vi "Equals.vi"(8 "error in (no error)":errorcluster, 10 "Other Parameter to Hardware Map in":refnum<class "Parameter to Hardware Map.lvclass">, 11 "Parameter to Hardware Map in":refnum<class "Parameter to Hardware Map.lvclass">) -> (0 "error out":errorcluster, 2 "Equal?":bool, 3 "Parameter to Hardware Map out":refnum<class "Parameter to Hardware Map.lvclass">)   [LabVIEW 2020, in "Parameter to Hardware Map.lvclass"]
doc: "Test if two maps are equal. Item order is not considered. Maps are considered equal if all elements of map_1 are included in map_2 and all elements of map_2 are included in map_1."
uses:
  Parameter to Hardware Map.lvclass
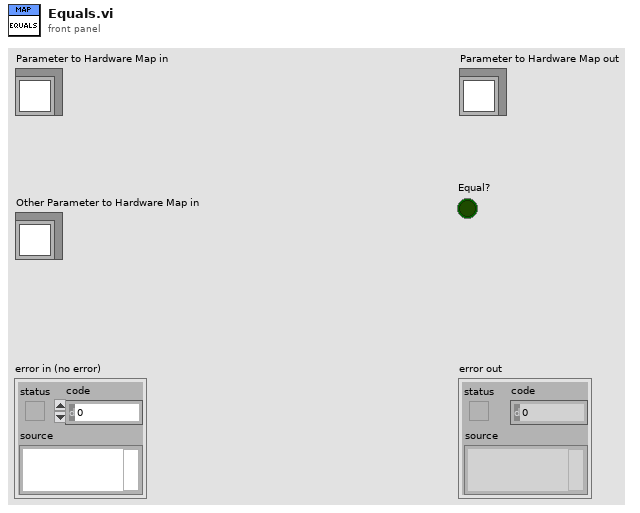
[diagram p1: front panel]
types:
  T1 = typedef "Parameter to Hardware Map.lvclass/Pair.ctl" = cluster{"key":string, "values":refnum<class "Generic Plugin.lvclass">[]}
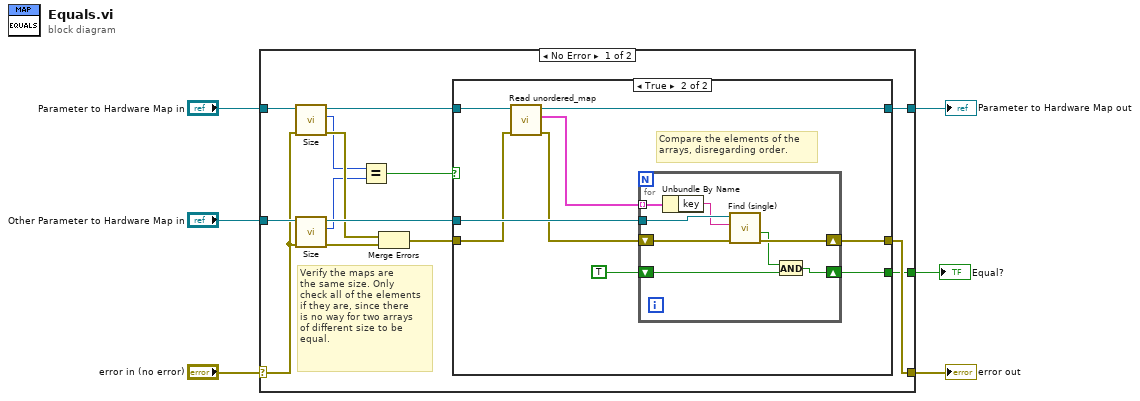
[diagram p0: block diagram]
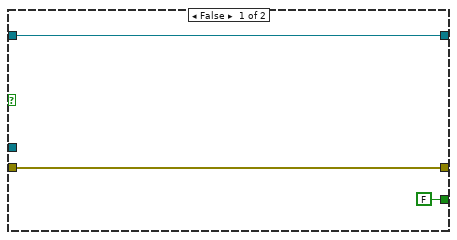
[diagram p2: hidden frame]
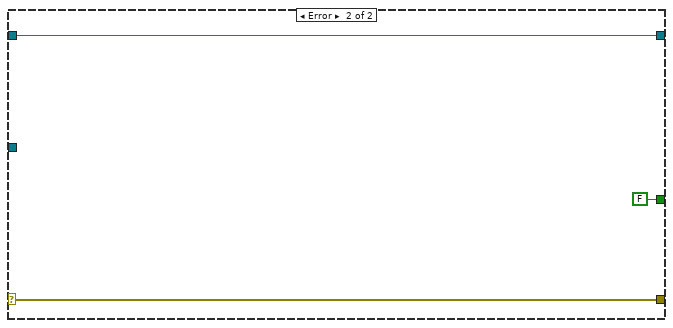
[diagram p3: hidden frame]
diagram:
  n1 = case shown="No Error" "error in (no error)" {
    selector: "error in (no error)" -> [w14 w43]
    tunnel: [w18 w43] -> w5
    tunnel: [w19 w42] -> w3
    tunnel: "Parameter to Hardware Map in" -> [w20 w42]
    tunnel: "Other Parameter to Hardware Map in" -> [w17 _]
    tunnel: [w7 FALSE] -> w1
    frame No Error {
      # "Verify the maps are\nthe same size. Only\ncheck all of the elements\nif they are, since there\nis no way for two arrays\nof different size to be\nequal."
      n2 = call "Size.vi"("error in (no error)"=w14, "Parameter to Hardware Map in"=w20) -> ("error out"=w12:errorcluster, "Size"=w11:i32, "Parameter to Hardware Map out"=w16:refnum<class "Parameter to Hardware Map.lvclass">)  [unwired: 7 in]
      n3 = call "Size.vi"("error in (no error)"=w14, "Parameter to Hardware Map in"=w17) -> ("error out"=w13:errorcluster, "Size"=w10:i32, "Parameter to Hardware Map out"=w15:refnum<class "Parameter to Hardware Map.lvclass">)  [unwired: 7 in]
      n4 = Equal?(x=w11, y=w10) -> (x = y?=w8:bool)
      n5 = Merge Errors(w12, w13) -> (w9:errorcluster)
      n6 = case shown="True" w8 {
        tunnel: [w23 w32] -> w19
        tunnel: [w22 w30] -> w18
        tunnel: w16 -> [w23 w28]
        tunnel: w15 -> [_ w27]
        tunnel: w9 -> [w22 w26]
        tunnel: [FALSE w24] -> w7
        frame False {
        }
        frame True {
          # "Compare the elements of the \narrays, disregarding order."
          n7 = call "Read unordered_map.vi"("error in (no error)"=w26, "Parameter to Hardware Map in"=w28) -> ("error out"=w25:errorcluster, "unordered_map"=w31:T1[], "Parameter to Hardware Map out"=w32:refnum<class "Parameter to Hardware Map.lvclass">)  [unwired: 7 in]
          n8 = for {
            tunnel: w31 -> [w38] mode=indexing
            shift-right: [w35] -> w30
            shift-left: w25 -> [w36]
            shift-right: [w33] -> w24
            shift-left: TRUE -> [w40]
            tunnel: w27 -> [w39]
            n9 = Unbundle By Name(w38) -> ("key"=w37:string)
            n10 = call "Find (single).vi"("error in (no error)"=w36, "Key"=w37, "Parameter to Hardware Map in"=w39) -> ("error out"=w35:errorcluster, "Found?"=w34:bool)  [unwired: 5 in, 2 out]
            n11 = And(x=w34, y=w40) -> (x .and. y?=w33:bool)
          }
        }
      }
    }
    frame Error {
    }
  }
  "error out" <- w5
  "Parameter to Hardware Map out" <- w3
  "Equal?" <- w1
